vi "Standard Setup.vi"(8 "error in (no error)":errorcluster, 10 "Previous CCD Config":T4={"EXPTIME"=1.0, "PREAMP"=enum."Gain 1", "READOUT_RATE"=enum."1 MHz", "EM_GAIN"=2, "VBIN"=1, "INITIAL_LINE"=1, "INITIAL_COLUMN"=1, "FINAL_LINE"=1024, "FINAL_COLUMN"=1024, "#FRAMES"=1, "#CUBES"=1, "TRIGGER_MODE"=enum."Internal", "HBIN"=1, "SHUTTER_TTL"=enum."TTL Low", "SHUTTER_MODE"=enum."Close", "SHUTTER_OPENING_TIME"=50, "SHUTTER_CLOSING_TIME"=50, "VERTICAL_SHIFT_SPEED"=3, "READ_MODE"=enum."Image", "FRAME_TRANSFER"=TRUE, "VERTICAL_CLOCK_VOLTAGE"=enum."0", "ACQUISITION_MODE"=enum."Kinetics", "AD_CHANNEL"=0, "EM_MODE"=enum."Electron Multiplying"}, 11 "CCDCamera in":refnum<class "CCDCamera.lvclass">) -> (0 "error out":errorcluster, 3 "CCDCamera out":refnum<class "CCDCamera.lvclass">)   [LabVIEW 2018, in "CCDCamera.lvclass"]
uses:
  CCDCamera.lvclass
  C:/Users/observer/Desktop/SPARC4_ACS/SPARC4_ACS/Simulated_CCD_Camera/Simulated_CCD_Camera.lvclass
  <userlib>/atmcd32d.llb/Shutter_mode typedef.ctl
  <userlib>/atmcd32d.llb/ReadMode_mode typedef.ctl
  <userlib>/atmcd32d.llb/AcquisitionMode_mode typedef.ctl
  Simulated_CCD_Camera/Simulated_CCD_Camera.lvclass/Simulated_CCD_Camera.ctl
  Simulated_CCD_Camera/Simulated_CCD_Camera.lvclass
  Interface/Interface.lvclass
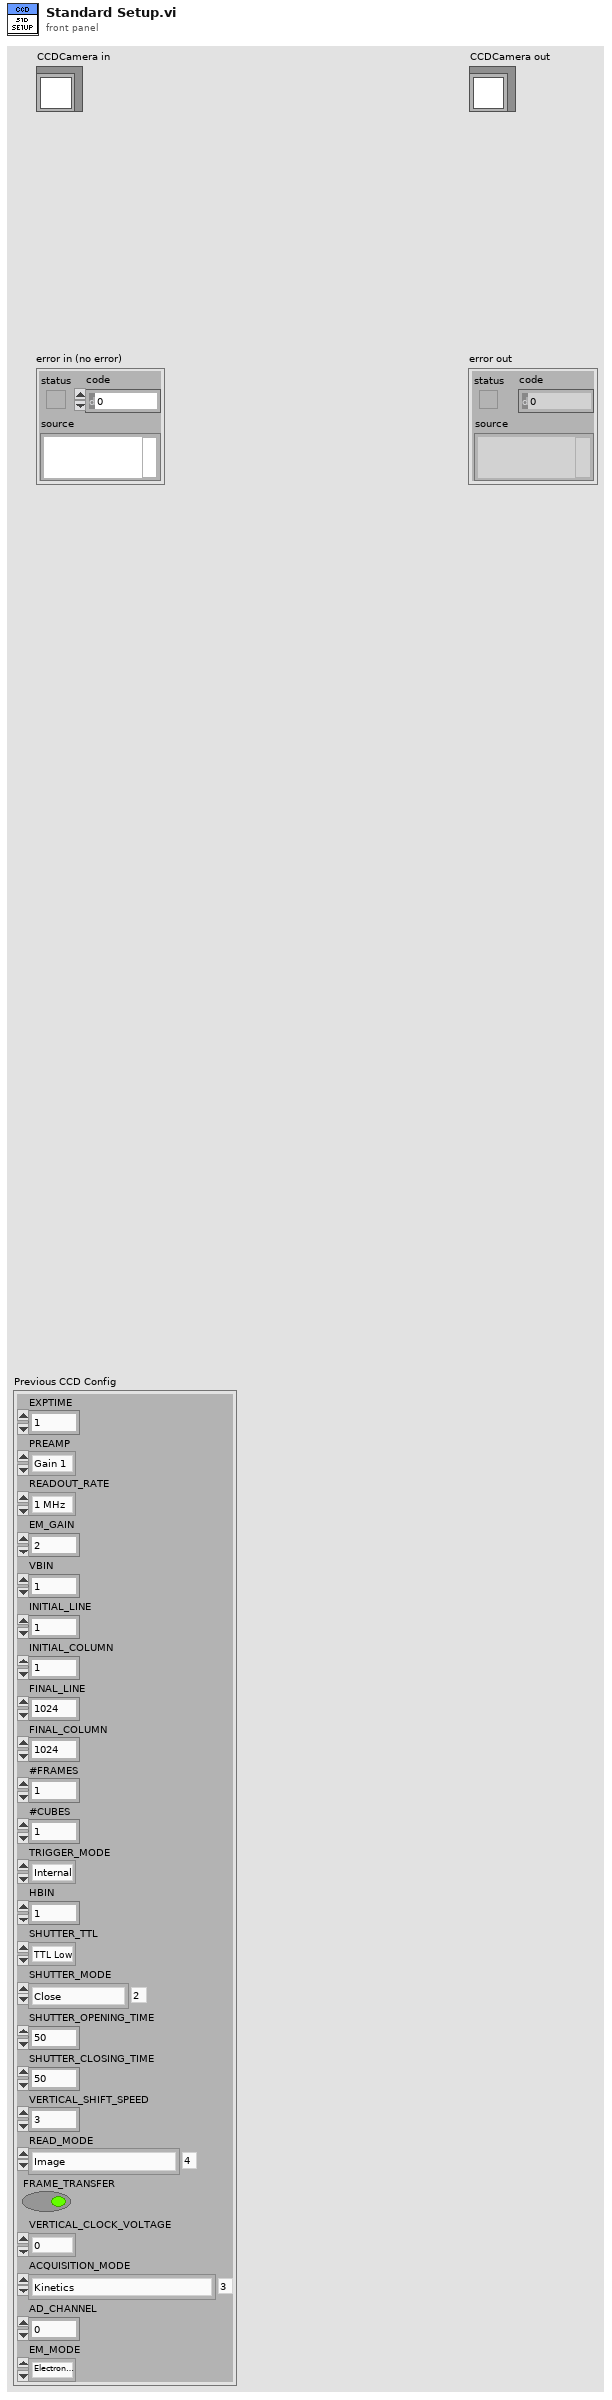
[diagram p1: front panel]
types:
  T1 = typedef "Shutter_mode typedef.ctl" = enum16{"Auto", "Open", "Close", "N/A (3)", "Open FVB Series", "Open Any Series"}
  T2 = typedef "ReadMode_mode typedef.ctl" = enum16{"Full Vertical Binning", "Multi-Track", "Random-Track", "Single-Track", "Image"}
  T3 = typedef "AcquisitionMode_mode typedef.ctl" = enum16{"Reserved (0)", "Single Scan", "Accumulate", "Kinetics", "Fast Kinetics", "Run Till Abort", "Reserved (6)", "Reserved (7)", "Reserved (8)", "Time Delayed Integration"}
  T4 = cluster{"EXPTIME":sgl, "PREAMP":enum16{"Gain 1", "Gain 2"}, "READOUT_RATE":enum16{"30 MHz", "20 MHz", "10 MHz", "1 MHz"}, "EM_GAIN":u16, "VBIN":u16, "INITIAL_LINE":u16, "INITIAL_COLUMN":u16, "FINAL_LINE":u16, "FINAL_COLUMN":u16, "#FRAMES":u32, "#CUBES":u32, "TRIGGER_MODE":enum16{"Internal", "External", "N/A", "N/A_1", "N/A_2", "N/A_3", "External Start"}, "HBIN":u16, "SHUTTER_TTL":enum16{"TTL Low", "TTL High"}, "SHUTTER_MODE":T1, "SHUTTER_OPENING_TIME":u16, "SHUTTER_CLOSING_TIME":u16, "VERTICAL_SHIFT_SPEED":u16, "READ_MODE":T2, "FRAME_TRANSFER":bool, "VERTICAL_CLOCK_VOLTAGE":enum16{"0", "+1", "+2", "+3", "+4"}, "ACQUISITION_MODE":T3, "AD_CHANNEL":u16, "EM_MODE":enum16{"Electron Multiplying", "Conventional"}}
  T5 = enum16{"Internal", "External", "N/A", "N/A_1", "N/A_2", "N/A_3", "External Start"}
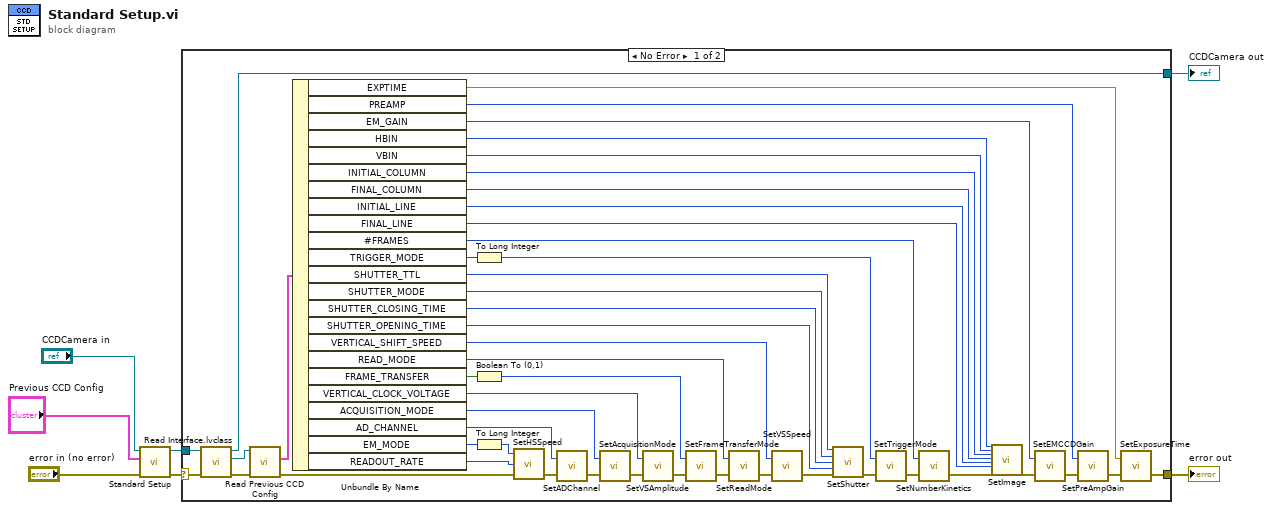
[diagram p0: block diagram]
diagram:
  n1 = call-parent "Standard Setup.vi"("error in (no error)"="error in (no error)", "Previous CCD Config"="Previous CCD Config", "CCDCamera in"="CCDCamera in") -> ("error out"=w4:errorcluster, "CCDCamera out"=w3:refnum<class "CCDCamera.lvclass">)  [unwired: 7 in]
  n2 = case shown="No Error" w4 {
    selector: w4 -> [w53 w55]
    tunnel: w3 -> [w54 w56]
    tunnel: [w8 w56] -> w2
    tunnel: [w9 w55] -> w1
    frame No Error {
      n3 = call "Read Interface.lvclass.vi"("error in (no error)"=w53, "Simulated_CCD_Camera in"=w54) -> ("error out"=w51:errorcluster, "Interface.lvclass"=w52:refnum<class "Interface.lvclass">, "Simulated_CCD_Camera out"=w8:refnum<class "CCDCamera.lvclass">)  [unwired: 7 in]
      n4 = call "Read Previous CCD Config.vi"("error in (no error)"=w51, "Interface in"=w52) -> ("error out"=w23:errorcluster, "Previous CCD Config"=w50:T4)  [unwired: 7 in, 1 out]
      n5 = Unbundle By Name(w50) -> ("EXPTIME"=w49:sgl, "PREAMP"=w47:enum16{"Gain 1", "Gain 2"}, "EM_GAIN"=w48:u16, "HBIN"=w36:u16, "VBIN"=w35:u16, "INITIAL_COLUMN"=w34:u16, "FINAL_COLUMN"=w33:u16, "INITIAL_LINE"=w32:u16, "FINAL_LINE"=w31:u16, "#FRAMES"=w45:u32, "TRIGGER_MODE"=w39:T5, "SHUTTER_TTL"=w30:enum16{"TTL Low", "TTL High"}, "SHUTTER_MODE"=w29:T1, "SHUTTER_CLOSING_TIME"=w28:u16, "SHUTTER_OPENING_TIME"=w27:u16, "VERTICAL_SHIFT_SPEED"=w41:u16, "READ_MODE"=w43:T2, "FRAME_TRANSFER"=w38:bool, "VERTICAL_CLOCK_VOLTAGE"=w44:enum16{"0", "+1", "+2", "+3", "+4"}, "ACQUISITION_MODE"=w46:T3, "AD_CHANNEL"=w42:u16, "EM_MODE"=w26:enum16{"Electron Multiplying", "Conventional"}, "READOUT_RATE"=w24:enum16{"30 MHz", "20 MHz", "10 MHz", "1 MHz"})
      n6 = To Long Integer(number=w39) -> (32bit integer=w40:i32)
      n7 = Boolean To (0,1)(Boolean=w38) -> (0, 1=w37:i16)
      n8 = To Long Integer(number=w26) -> (32bit integer=w25:i32)
      n9 = call <userlib>:"SetHSSpeed.vi"("error in (no error)"=w23, "index"=w24, "type"=w25) -> ("error out"=w22:errorcluster)  [unwired: 1 in, 1 out]
      n10 = call <userlib>:"SetADChannel.vi"("error in (no error)"=w22, "channel"=w42) -> ("error out"=w21:errorcluster)  [unwired: 1 out]
      n11 = call <userlib>:"SetAcquisitionMode.vi"("error in (no error)"=w21, "mode"=w46) -> ("error out"=w20:errorcluster)  [unwired: 1 out]
      n12 = call <userlib>:"SetVSAmplitude.vi"("error in (no error)"=w20, "amplitude"=w44) -> ("error out"=w19:errorcluster)  [unwired: 1 out]
      n13 = call <userlib>:"SetFrameTransferMode.vi"("error in (no error)"=w19, "mode"=w37) -> ("error out"=w18:errorcluster)  [unwired: 1 out]
      n14 = call <userlib>:"SetReadMode.vi"("error in (no error)"=w18, "mode"=w43) -> ("error out"=w17:errorcluster)  [unwired: 1 out]
      n15 = call <userlib>:"SetVSSpeed.vi"("error in (no error)"=w17, "index"=w41) -> ("error out"=w16:errorcluster)  [unwired: 1 out]
      n16 = call <userlib>:"SetShutter.vi"("type"=w30, "mode"=w29, "closingtime"=w28, "openingtime"=w27, "error in (no error)"=w16) -> ("error out"=w15:errorcluster)  [unwired: 9 in, 1 out]
      n17 = call <userlib>:"SetTriggerMode.vi"("error in (no error)"=w15, "mode"=w40) -> ("error out"=w14:errorcluster)  [unwired: 1 out]
      n18 = call <userlib>:"SetNumberKinetics.vi"("error in (no error)"=w14, "number"=w45) -> ("error out"=w13:errorcluster)  [unwired: 1 out]
      n19 = call <userlib>:"SetImage.vi"("hbin"=w36, "vbin"=w35, "hstart"=w34, "hend"=w33, "vstart"=w32, "vend"=w31, "error in (no error)"=w13) -> ("error out"=w12:errorcluster)  [unwired: 19 in, 1 out]
      n20 = call <userlib>:"SetEMCCDGain.vi"("error in (no error)"=w12, "gain"=w48) -> ("error out"=w11:errorcluster)  [unwired: 1 out]
      n21 = call <userlib>:"SetPreAmpGain.vi"("error in (no error)"=w11, "index"=w47) -> ("error out"=w10:errorcluster)  [unwired: 1 out]
      n22 = call <userlib>:"SetExposureTime.vi"("error in (no error)"=w10, "time"=w49) -> ("error out"=w9:errorcluster)  [unwired: 1 out]
    }
    frame Error {
    }
  }
  "error out" <- w1
  "CCDCamera out" <- w2
